vi "force_control.vi"(2 "Goal position in":sgl[][](array[numeric])) -> (16 "Goal position out":sgl[][](array[numeric]))   [LabVIEW 2013]
uses:
  <vilib>/Analysis/Matrix/Datatypes/RealMatrix.ctl
  <vilib>/Analysis/baseanly.llb/A x Vector.vi
  <vilib>/Analysis/baseanly.llb/Real Inverse Matrix.vi
  <vilib>/Analysis/NI_AALBase.lvlib
  <vilib>/Analysis/Matrix/NI_Matrix.lvlib
panel:
  out "Force In":T1
  out "Probe Output":T1
  out "Transformed Goal Pts":T1
  out "Accelerometer In":T1
  in  "Gain Matrix (Kp)":T1=[[0.0, 0.0, 110000.0], [0.0, 0.0, 0.0], [0.0, 0.0, 0.0]]
  in  "Force Setpoints":T1=[[0.0, 0.0, 0.0245], [0.0, 0.0, 0.0]]
  in  "Surface to ASAP Rotation Matrix":T1=[[-0.94340685160565, -0.32848364418107, 0.045629024195576, 9068.109203025148], [0.283835534373385, -0.870906704437691, -0.401196836468652, -24863.68471797479], [0.171525221966017, -0.365540705901551, 0.914854682754865, -63368.71671959403], [0.0, 0.0, 0.0, 1.0]]
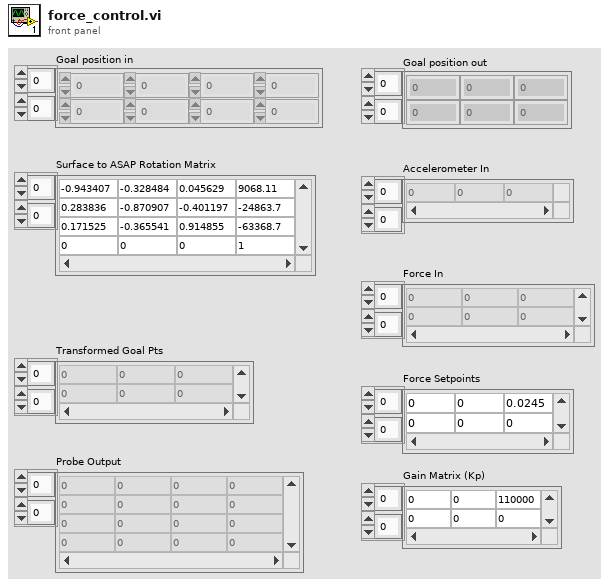
[diagram p1: front panel]
types:
  T1 = typedef "NI_Matrix.lvlib/RealMatrix.ctl" = dbl[][]
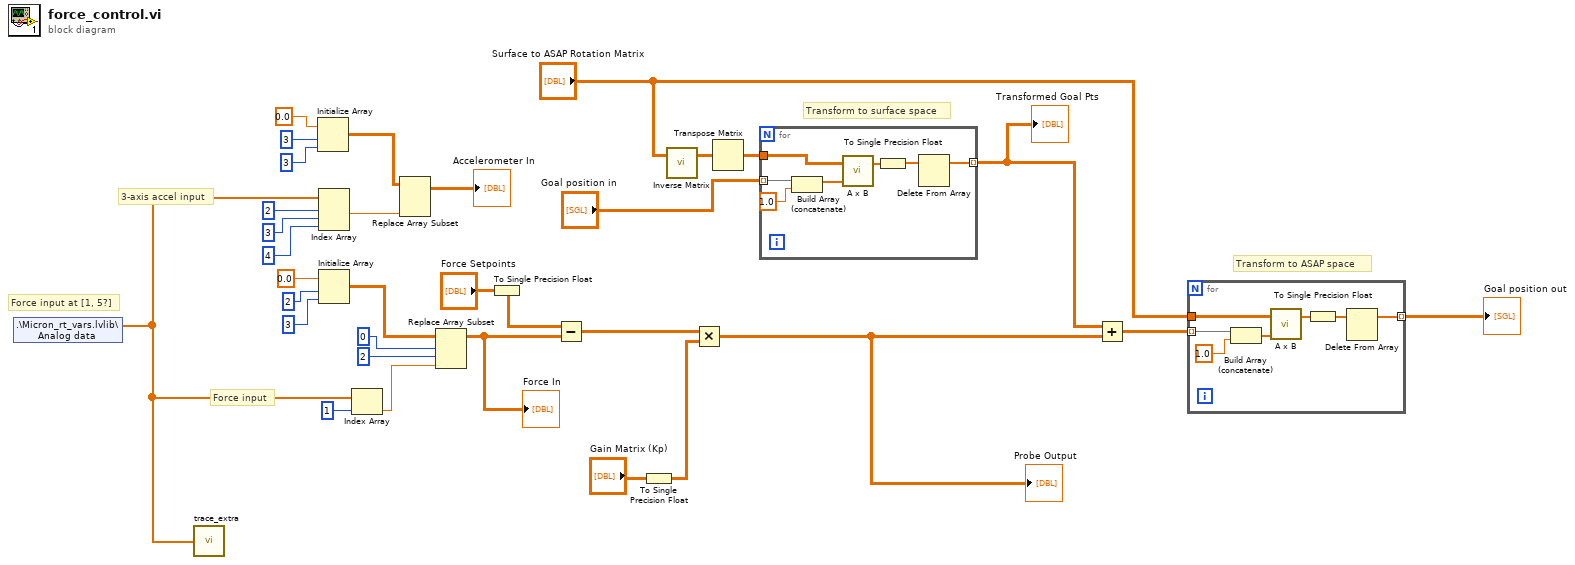
[diagram p0: block diagram]
diagram:
  # "Force input"
  # "Transform to surface space"
  # "Transform to ASAP space"
  # "Force input at [1, 5?]"
  # "3-axis accel input"
  n1 = shared-variable ".\\Micron_rt_vars.lvlib\\Analog data"() -> (w10:sgl[])  [unwired: 1 in, 1 out]
  n2 = call "trace_extra.vi"("Extra trace data"=w10) -> ()  [unwired: 1 in]
  n3 = Initialize Array(sgl 0.0, 3, 3) -> (w4:sgl[][])
  n4 = Index Array(array=w10, index #1=2, index #2=3, index #3=4) -> (element #1=w25:sgl)  [unwired: 2 out]
  n5 = Initialize Array(sgl 0.0, 2, 3) -> (w3:sgl[][])
  n6 = Index Array(array=w10, index=1) -> (element=w31:sgl)
  n7 = Replace Array Subset(array=w4, new element=w25) -> (→"Accelerometer In":T1)  [unwired: 2 in]
  n8 = Replace Array Subset(array=w3, new element=w31, index (row)=0, index (col)=2) -> (w1:sgl[][])
  "Force In" <- w1
  n9 = To Single Precision Float(number="Force Setpoints") -> (single precision float=w18:sgl[][])
  n10 = Subtract ("Subtract.vi")(x=w18, y=w1) -> (x-y=w2:sgl[][])
  n11 = To Single Precision Float(number="Gain Matrix (Kp)") -> (single precision float=w29:sgl[][])
  n12 = call-poly <vilib>:"Inverse Matrix.vi"("Input Matrix"="Surface to ASAP Rotation Matrix") -> ("Inverse Matrix"=w17:T1)  [unwired: 1 in, 1 out]
  n13 = Multiply ("Multiply.vi")(x=w2, y=w29) -> (x*y=w8:sgl[][])
  "Probe Output" <- w8
  n14 = Transpose Matrix(1:w17) -> (0:w16:T1)
  n15 = for {
    tunnel: "Goal position in" -> [w35] mode=indexing
    tunnel: w16 -> [w37]
    tunnel: [w36] -> w14 mode=indexing
    n16 = Build Array (concatenate)(w35, sgl 1.0) -> (w33:sgl[])
    n17 = call-poly <vilib>:"A x B.vi"("Vector"=w33, "A"=w37) -> ("A x Vector"=w38:dbl[])  [unwired: 1 out]
    n18 = To Single Precision Float(number=w38) -> (single precision float=w39:sgl[])
    n19 = Delete From Array(array=w39) -> (array with subset deleted=w36:sgl[])  [unwired: 2 in, 1 out]
  }
  "Transformed Goal Pts" <- w14
  n20 = Add ("Add.vi")(x=w14, y=w8) -> (x+y=w26:sgl[][])
  n21 = for {
    tunnel: w26 -> [w42] mode=indexing
    tunnel: "Surface to ASAP Rotation Matrix" -> [w41]
    tunnel: [w40] -> w27 mode=indexing
    n22 = Build Array (concatenate)(w42, sgl 1.0) -> (w45:sgl[])
    n23 = call-poly <vilib>:"A x B.vi"("Vector"=w45, "A"=w41) -> ("A x Vector"=w43:dbl[])  [unwired: 1 out]
    n24 = To Single Precision Float(number=w43) -> (single precision float=w46:sgl[])
    n25 = Delete From Array(array=w46) -> (array with subset deleted=w40:sgl[])  [unwired: 2 in, 1 out]
  }
  "Goal position out" <- w27
